vi "RCM Go to Case MHLC.vi"(8 "error in (no error)":errorcluster, 10 "Data":variant, 11 "Message Log in":refnum<class "Message Log.lvclass">) -> (0 "error out":errorcluster, 3 "Message Log out":refnum<class "Message Log.lvclass">)   [LabVIEW 2017, in "Message Log.lvclass"]
doc: "Show the selected MHL Case the front panel of the selected Worker's Main VI"
uses:
  Message Log.lvclass
  Message Log.lvclass/Message Log.ctl
  rql_RCM Go to Case.ctl
  Listbox Selection.ctl
  <vilib>/Utility/miscctls.llb/LVRowAndColumnTypeDef.ctl
  rsp_Go to MHL Case.ctl
  Common VIs/Message Log ID.ctl
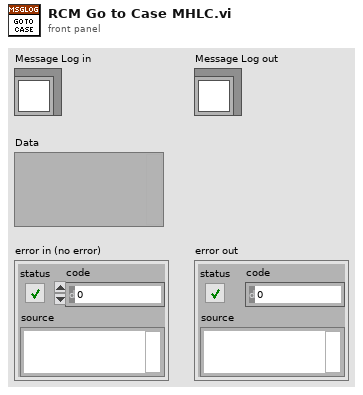
[diagram p1: front panel]
types:
  T1 = typedef "Message Log.lvclass/rql_RCM Go to Case.ctl" = cluster{"Listbox Selection":T2}
  T2 = typedef "Message Log.lvclass/Listbox Selection.ctl" = cluster{"Cell Position":T3, "Row":string[]}
  T3 = typedef "LVRowAndColumnTypeDef.ctl" = cluster{"Row":i32, "Column":i32}
  T4 = typedef "Message Log.lvclass/rsp_Go to MHL Case.ctl" = cluster{"Message Log ID":T5, "Worker ID":string, "Case Name":string}
  T5 = typedef "Message Log ID.ctl" = cluster{"Head Worker ID":string, "IP Address":string}
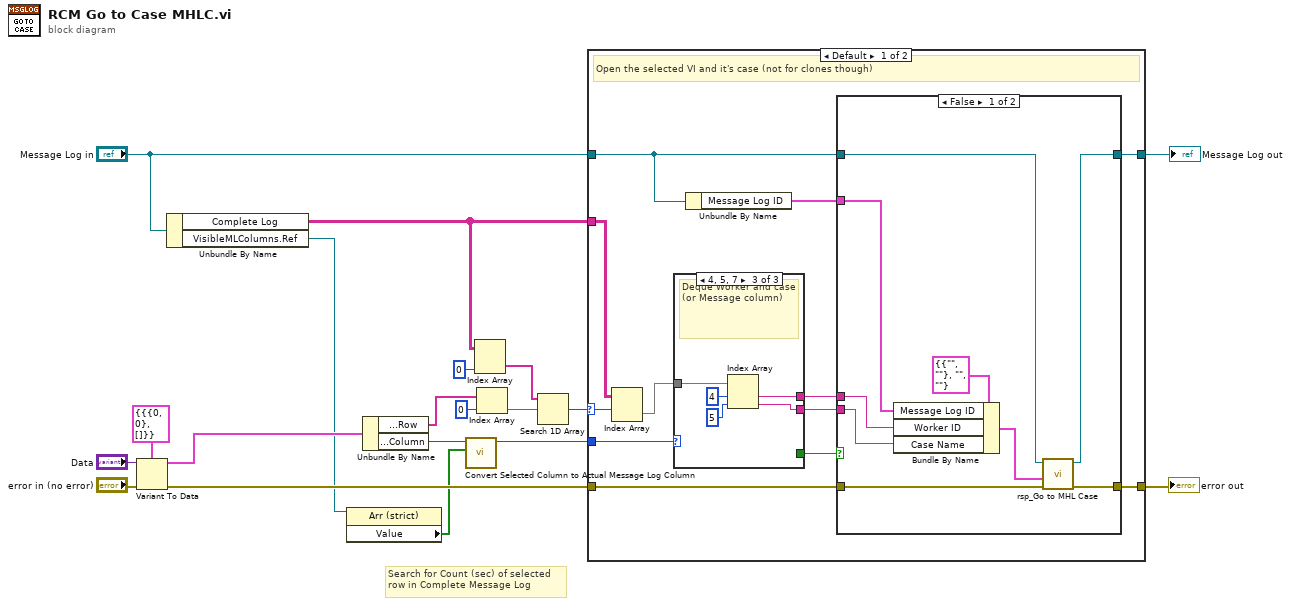
[diagram p0: block diagram]
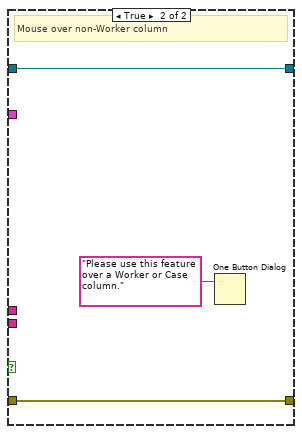
[diagram p2: hidden frame]
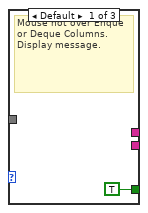
[diagram p3: hidden frame]
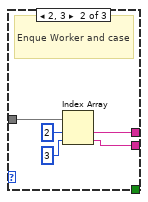
[diagram p4: hidden frame]
diagram:
  # "Search for Count (sec) of selected\nrow in Complete Message Log"
  n1 = Variant To Data(error in="error in (no error)", type=T1 {"Listbox Selection"={"Cell Position"={"Row"=0, "Column"=0}, "Row"=[]}} ("Data"), Variant="Data") -> (data=w10:T1, error out=w9:errorcluster)
  n2 = Unbundle By Name("Message Log in") -> ("Complete Log"=w4:string[][], "VisibleMLColumns.Ref"=w6:refnum<vi>)
  n3 = property class="Arr (strict)"(reference=w6) -> ("Value"=w5:bool[])  [unwired: 1 in, 2 out]
  n4 = Unbundle By Name(w10) -> ("Listbox Selection.Row"=w16:string[], "Listbox Selection.Cell Position.Column"=w11:i32)
  n5 = call "Convert Selected Column to Actual Message Log Column.vi"("Visible ML Columns"=w5, "Selected Column"=w11) -> ("Actual Column"=w8:i32)  [unwired: 9 in]
  n6 = Index Array(array=w4, index (col)=0 ("disabled index (col)")) -> (element=w12:string[])  [unwired: 1 in]
  n7 = Index Array(array=w16, index=0) -> (element=w13:string)
  n8 = Search 1D Array(1D array=w12, element=w13) -> (index of element=w3:i32)  [unwired: 1 in]
  n9 = case shown="Default" w3 {
    selector: w3 -> [w28 _]
    tunnel: [w26 w56] -> w7
    tunnel: w9 -> [w25 w56]
    tunnel: w4 -> [w31 _]
    tunnel: w8 -> [w30 _]
    tunnel: [w23 w55] -> w1
    tunnel: "Message Log in" -> [w24 w55]
    frame Default {
      # "Open the selected VI and it's case (not for clones though)"
      n10 = Index Array(array=w31, index (row)=w28) -> (element=w29:string[])  [unwired: 1 in]
      n11 = case shown="4, 5, 7" w30 {
        tunnel: w29 -> [_ w48 w53]
        tunnel: [_ w47 w52] -> w21
        tunnel: [TRUE _ _] -> w27
        tunnel: [_ w45 w51] -> w20
        frame Default {
          # "Mouse not over Enque or Deque Columns.\nDisplay message."
        }
        frame 2, 3 {
          # "Enque Worker and case"
          n12 = Index Array(array=w48, index #1=2 ("index"), index #2=3 ("index")) -> (element #1=w47:string, element #2=w45:string)
        }
        frame 4, 5, 7 {
          # "Deque Worker and case (or Message column)"
          n13 = Index Array(array=w53, index #1=4 ("index"), index #2=5 ("index")) -> (element #1=w52:string, element #2=w51:string)
        }
      }
      n14 = Unbundle By Name(w24) -> ("Message Log ID"=w22:T5)
      n15 = case shown="False" w27 {
        tunnel: [w35 w42] -> w26
        tunnel: w25 -> [w36 w42]
        tunnel: w24 -> [w38 w41]
        tunnel: [w37 w41] -> w23
        tunnel: w22 -> [w34 _]
        tunnel: w21 -> [w33 _]
        tunnel: w20 -> [w32 _]
        frame False {
          n16 = Bundle By Name(cluster=T4 {"Message Log ID"={"Head Worker ID"="", "IP Address"=""}, "Worker ID"="", "Case Name"=""} ("Data in"), "Message Log ID"=w34, "Worker ID"=w33, "Case Name"=w32) -> (w39:T4)
          n17 = call "rsp_Go to MHL Case.vi"("error in"=w36, "Data in"=w39, "Message Log in"=w38) -> ("error out"=w35:errorcluster, "dup Message Log out"=w37:refnum<class "Message Log.lvclass">)  [unwired: 7 in]
        }
        frame True {
          # "Mouse over non-Worker column"
          n18 = One Button Dialog(message="Please use this feature over a Worker or Case column.") -> ()  [unwired: 1 in, 1 out]
        }
      }
    }
    frame -1 {
      # "Can't find Row in complete message log\nPossible that this row doesn't exist in the Complete message log any longer. Do nothing"
    }
  }
  "Message Log out" <- w1
  "error out" <- w7
